vi "emi_Movement simple.vi"(0 "Position(0)":dbl, 5 "Time(self timed)":dbl=-1.0, 11 "error in (no error)":errorcluster) -> (4 "Position Out":dbl, 6 "Velosity Out":dbl, 8 "Acceleration Out":dbl, 15 "error out":errorcluster)   [LabVIEW 2010]
doc: "Calculate instance position, velosity and Acceleration based on the previous thre positions and their time difference.\n\nReentrant subroutine\n\nIgnores errors."
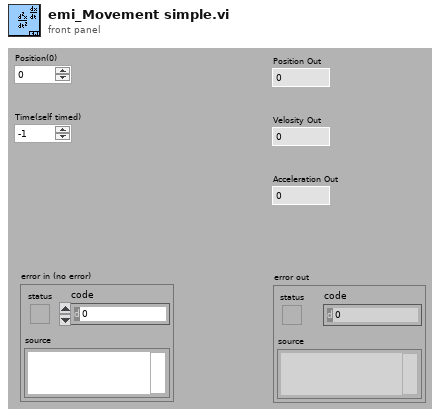
[diagram p1: front panel]
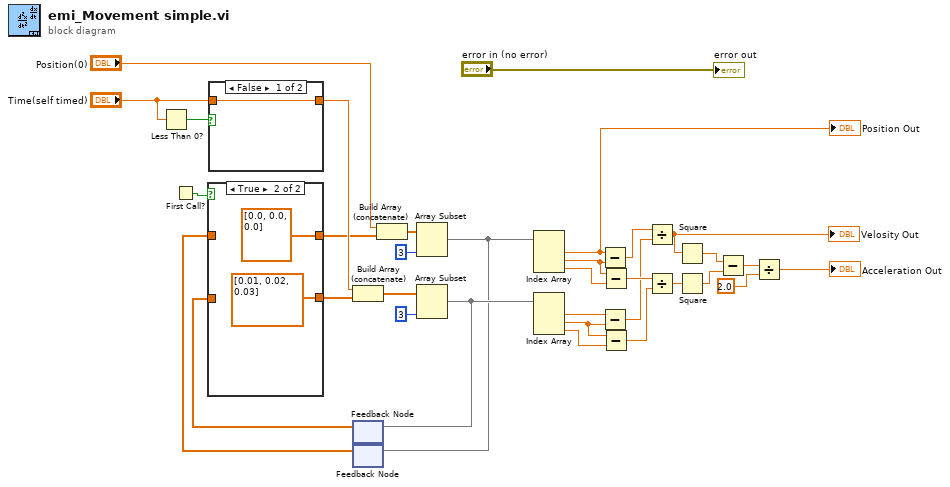
[diagram p0: block diagram]
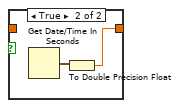
[diagram p2: hidden frame]
diagram:
  n1 = Less Than 0?(x="Time(self timed)") -> (x < 0?=w13:bool)
  n2 = First Call?() -> (First Call?: T/F=w4:bool)
  n3 = case shown="False" w13 {
    tunnel: "Time(self timed)" -> [w34 _]
    tunnel: [w34 w35] -> w15
    frame False {
    }
    frame True {
      n4 = Get Date/Time In Seconds() -> (seconds since 1Jan1904=w36:timestamp)
      n5 = To Double Precision Float(number=w36) -> (double precision float=w35:dbl)
    }
  }
  n6 = feedback #1() -> (w12:dbl[])  [unwired: 1 in]
  n7 = feedback #2() -> (w8:dbl[])  [unwired: 1 in]
  n8 = case shown="True" w4 {
    tunnel: w8 -> [w38 _]
    tunnel: [w38 dbl[] [0.0, 0.0, 0.0]] -> w9
    tunnel: [w37 dbl[] [0.01, 0.02, 0.03]] -> w11
    tunnel: w12 -> [w37 _]
    frame False {
    }
    frame True {
    }
  }
  n9 = Build Array (concatenate)(w15, w11) -> (w2:dbl[])
  n10 = Build Array (concatenate)("Position(0)", w9) -> (w5:dbl[])
  n11 = Array Subset(array=w5, length=3) -> (w1:dbl[])  [unwired: 1 in]
  n12 = feedback-in #2(w1) -> ()
  n13 = Array Subset(array=w2, length=3) -> (w26:dbl[])  [unwired: 1 in]
  n14 = feedback-in #1(w26) -> ()
  n15 = Index Array(array=w1) -> (element #1=w18:dbl, element #2=w19:dbl, element #3=w20:dbl)  [unwired: 3 in]
  "Position Out" <- w18
  n16 = Index Array(array=w26) -> (element #1=w25:dbl, element #2=w16:dbl, element #3=w17:dbl)  [unwired: 3 in]
  n17 = Subtract(x=w18, y=w19) -> (x-y=w21:dbl)
  n18 = Subtract(x=w25, y=w16) -> (x-y=w22:dbl)
  n19 = Subtract(x=w19, y=w20) -> (x-y=w23:dbl)
  n20 = Subtract(x=w16, y=w17) -> (x-y=w24:dbl)
  n21 = Divide(x=w21, y=w22) -> (x/y=w27:dbl)
  "Velosity Out" <- w27
  n22 = Divide(x=w23, y=w24) -> (x/y=w28:dbl)
  n23 = Square(x=w27) -> (x^2=w29:dbl)
  n24 = Square(x=w28) -> (x^2=w30:dbl)
  n25 = Subtract(x=w29, y=w30) -> (x-y=w31:dbl)
  n26 = Divide(x=w31, y=2.0) -> (x/y=→"Acceleration Out":dbl)
  "error out" <- "error in (no error)"
